vi "NotZero.vi"(1 "Station to deliver":u16(ring) items=["", "A", "B", "C"], 2 "Numbers of Bottles":u16(ring) items=["0", "100", "200", "300", "400", "500"]) -> (0 "True":bool)   [LabVIEW 2020]
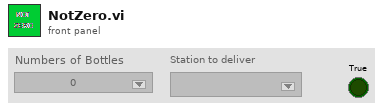
[diagram p1: front panel]
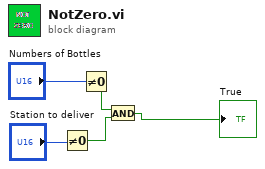
[diagram p0: block diagram]
diagram:
  n1 = Not Equal To 0?(x="Station to deliver") -> (x != 0?=w3:bool)
  n2 = Not Equal To 0?(x="Numbers of Bottles") -> (x != 0?=w2:bool)
  n3 = And(x=w2, y=w3) -> (x .and. y?=→"True":bool)
